vi "RT Loop - Watchdog.vi"(11 "Message Queue":refnum<queue>) -> ()   [LabVIEW 2022 SP3]
uses:
  support/Message Queue/Message Cluster.ctl
  <vilib>/RTwatchdog.llb/Watchdog expiration actions.ctl
  <vilib>/RTwatchdog.llb/Watchdog status enum.ctl
  Globals/Global - Configuration Options.vi
  support/Message Queue/Message Queue.lvlib
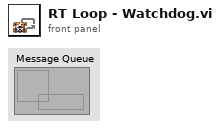
[diagram p1: front panel]
types:
  T1 = typedef "Watchdog status enum.ctl" = enum16{"disabled", "expired", "running"}
  T2 = typedef "Watchdog expiration actions.ctl" = cluster{"reset":bool, "occurrence":bool, "trigger protocol":enum16{"active high", "active low", "open collector"}, "trigger line":enum16{"none", "line 0", "line 1", "line 2", "line 3", "line 4", "line 5", "line 6", "line 7", "SMB line 0"}, "disable watchdog on VI exit":bool}
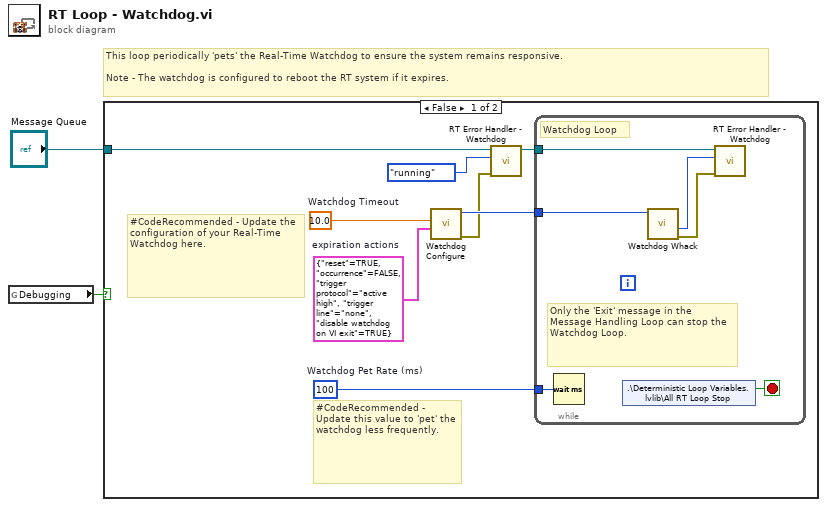
[diagram p0: block diagram]
diagram:
  # "This loop periodically 'pets' the Real-Time Watchdog to ensure the system remains responsive. \n\nNote - The watchdog is configured to reboot the RT system if it expires."
  n1 = global read "Global - Configuration Options.vi" "Debugging"() -> (w1:bool)
  n2 = case shown="False" w1 {
    tunnel: "Message Queue" -> [w10 _]
    frame False {
      w4 = u32 100  # Watchdog Pet Rate (ms)
      w5 = T2 {"reset"=TRUE, "occurrence"=FALSE, "trigger protocol"=enum."active high", "trigger line"=enum."none", "disable watchdog on VI exit"=TRUE}  # expiration actions
      w6 = 10.0  # Watchdog Timeout
      # "#CodeRecommended - Update the configuration of your Real-Time Watchdog here."
      # "#CodeRecommended - Update this value to 'pet' the watchdog less frequently."
      n3 = call <vilib>:"Watchdog Configure.vi"("expiration actions"=w5, "timeout (1 sec)"=w6) -> ("error out"=w7:errorcluster, "watchdogID"=w8:u32)  [unwired: 2 in, 2 out]
      n4 = call "RT Error Handler - Watchdog.vi"("error in (no error)"=w7, "watchdog status"=Watchdog_status_enum."running", "Message Queue"=w10) -> ("dup Message Queue"=w9:refnum<queue>)  [unwired: 8 in]
      n5 = while {
        tunnel: w9 -> [w16]
        tunnel: w8 -> [w14]
        tunnel: w4 -> [w15]
        stop <- w11 stop-if-true
        # "Only the 'Exit' message in the  Message Handling Loop can stop the Watchdog Loop."
        # "Watchdog Loop"
        n6 = Wait (ms)(milliseconds to wait=w15) -> ()  [unwired: 1 out]
        n7 = shared-variable ".\\Deterministic Loop Variables.lvlib\\All RT Loop Stop"() -> (w11:bool)  [unwired: 1 in, 1 out]
        n8 = call <vilib>:"Watchdog Whack.vi"("watchdogID in"=w14) -> ("error out"=w13:errorcluster, "watchdog status"=w12:T1)  [unwired: 4 in, 1 out]
        n9 = call "RT Error Handler - Watchdog.vi"("error in (no error)"=w13, "watchdog status"=w12, "Message Queue"=w16) -> ()  [unwired: 8 in, 1 out]
      }
    }
    frame True {
      # "Do not enable the watchdog when debugging."
    }
  }
